vi "Labview_FFT_Linear_Tianyi.vi"(0 "Channel A":u16[](array[numeric]), 5 "Channel B":u16[](array[numeric]), 7 "Resample Array":i32[](array[numeric]), 9 "Input Parameters":T1={"Points Per A-Scan"=0, "A-Scans per B-Scan"=0, "Voltage Range"=4.0, "Card Resolution (bits)"=16}) -> (4 "Int B-Scan Channel A":sgl[][](array[numeric]), 6 "Phase B-Scan Channel A":sgl[][](array[numeric]), 10 "Int B-Scan Channel B":sgl[][](array[numeric]), 13 "Raw B":u16[][](array[numeric]), 14 "Raw A":u16[][](array[numeric]), 15 "Phase B-Scan Channel B":sgl[][](array[numeric]))   [LabVIEW 2012]
uses:
  Type Defs/OCT Imaging Parameters Cluster.ctl
  <vilib>/Analysis/4window.llb/Hanning Window (DBL).vi
  <vilib>/Analysis/2dsp.llb/Real FFT.vi
  <vilib>/Analysis/NI_AALPro.lvlib
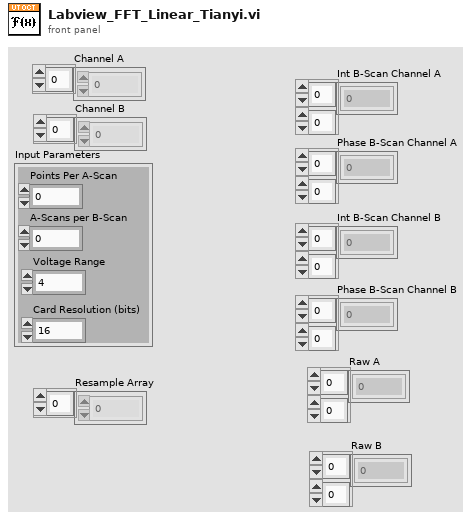
[diagram p1: front panel]
types:
  T1 = typedef "OCT Imaging Parameters Cluster.ctl" = cluster{"Points Per A-Scan":i32, "A-Scans per B-Scan":i32, "Voltage Range":sgl, "Card Resolution (bits)":u16}
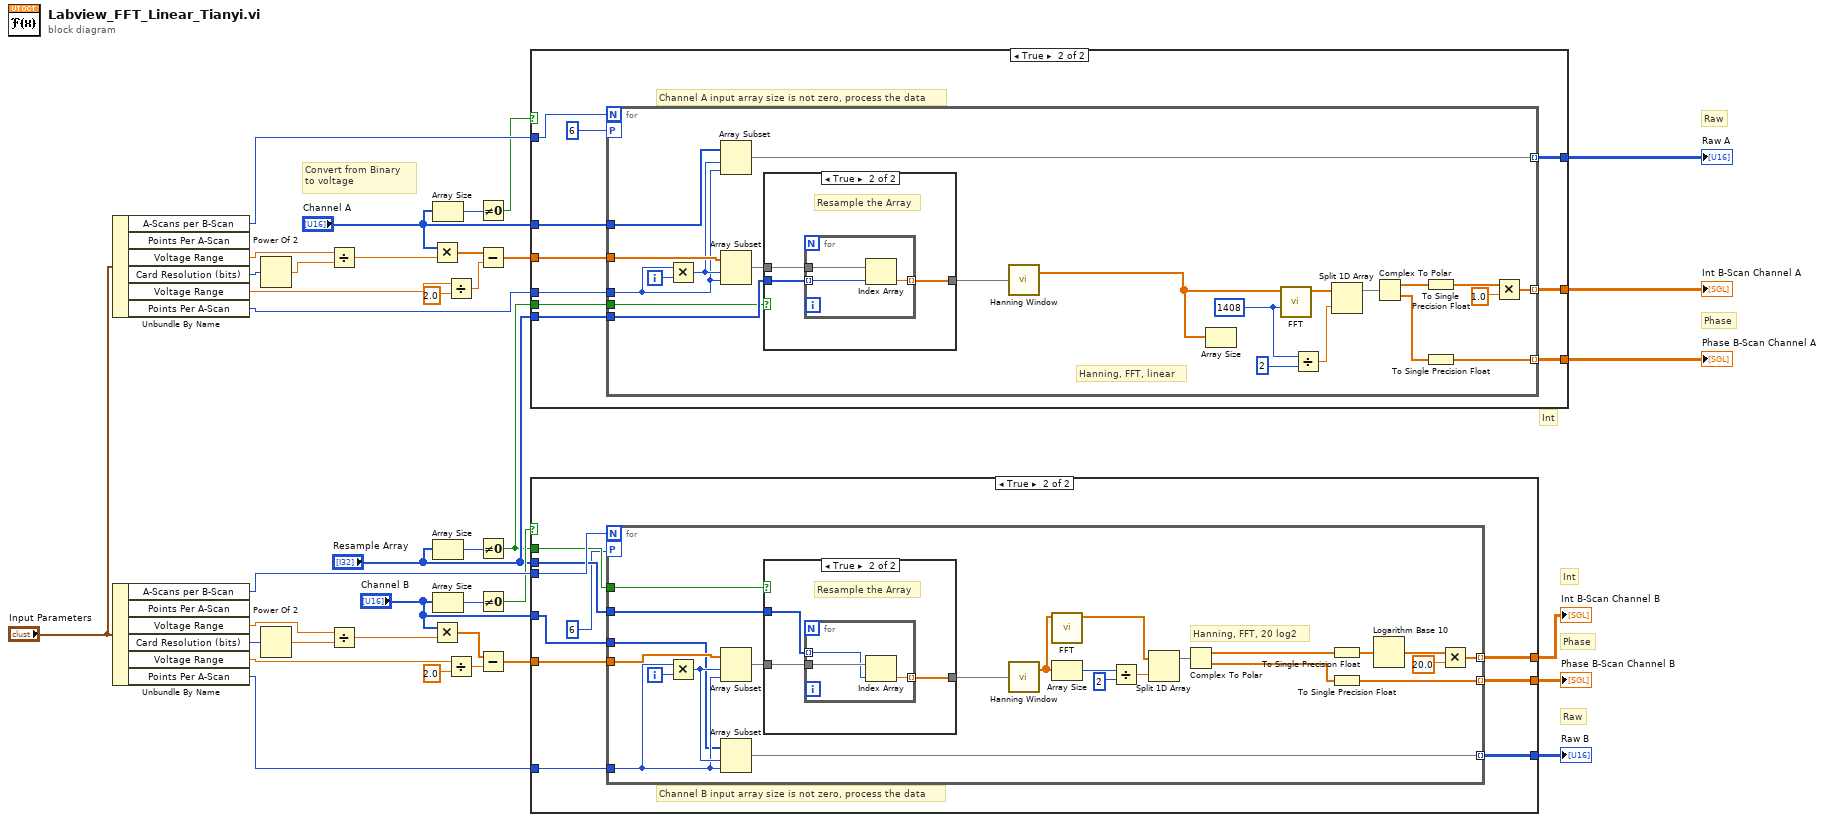
[diagram p0: block diagram]
diagram:
  # "Raw"
  # "Raw"
  # "Convert from Binary \nto voltage"
  # "Phase"
  # "Int"
  # "Phase"
  # "Int"
  n1 = Unbundle By Name("Input Parameters") -> ("A-Scans per B-Scan"=w36:i32, "Voltage Range"=w32:sgl, "Card Resolution (bits)"=w33:u16, "Voltage Range"=w30:sgl, "Points Per A-Scan"=w28:i32)  [unwired: 1 out]
  n2 = Unbundle By Name("Input Parameters") -> ("A-Scans per B-Scan"=w19:i32, "Voltage Range"=w23:sgl, "Card Resolution (bits)"=w22:u16, "Voltage Range"=w25:sgl, "Points Per A-Scan"=w27:i32)  [unwired: 1 out]
  n3 = Power Of 2(x=w33) -> (2^x=w35:dbl)
  n4 = Power Of 2(x=w22) -> (2^x=w20:dbl)
  n5 = Divide(x=w32, y=w35) -> (x/y=w34:dbl)
  n6 = Divide(x=w23, y=w20) -> (x/y=w21:dbl)
  n7 = Multiply(x="Channel A", y=w34) -> (x*y=w38:dbl[])
  n8 = Multiply(x="Channel B", y=w21) -> (x*y=w17:dbl[])
  n9 = Array Size(array="Channel A") -> (size(s)=w15:i32)
  n10 = Array Size(array="Resample Array") -> (size(s)=w3:i32)
  n11 = Array Size(array="Channel B") -> (size(s)=w13:i32)
  n12 = Divide(x=w30, y=sgl 2.0) -> (x/y=w31:sgl)
  n13 = Divide(x=w25, y=sgl 2.0) -> (x/y=w24:sgl)
  n14 = Not Equal To 0?(x=w15) -> (x != 0?=w14:bool)
  n15 = Subtract(x=w38, y=w31) -> (x-y=w37:dbl[])
  n16 = Not Equal To 0?(x=w3) -> (x != 0?=w1:bool)
  n17 = Not Equal To 0?(x=w13) -> (x != 0?=w12:bool)
  n18 = Subtract(x=w17, y=w24) -> (x-y=w18:dbl[])
  n19 = case shown="True" w14 {
    tunnel: w37 -> [_ w48]
    tunnel: [_ w47] -> w11
    tunnel: w36 -> [_ w46]
    tunnel: w28 -> [_ w45]
    tunnel: [_ w44] -> w8
    tunnel: "Channel A" -> [_ w43]
    tunnel: [_ w42] -> w6
    tunnel: "Resample Array" -> [_ w41]
    tunnel: w1 -> [_ w40]
    frame False {
      # "Channel A array size is zero, don't process data"
    }
    frame True {
      # "Channel A input array size is not zero, process the data"
      n20 = for {
        N: w46 -> [_]
        tunnel: w48 -> [w70]
        tunnel: w45 -> [w59]
        tunnel: [w66] -> w47 mode=indexing
        tunnel: [w62] -> w44 mode=indexing
        tunnel: w43 -> [w61]
        tunnel: [w58] -> w42 mode=indexing
        tunnel: w41 -> [w57]
        tunnel: w40 -> [w54]
        workers-P: 6 -> [_]
        i -> [w69]
        w49 = 1408 ("FFT size")
        # "Hanning, FFT, linear"
        n21 = Multiply(x=w59, y=w69) -> (x*y=w60:i32)
        n22 = Array Subset(array=w61, index=w60, length=w59) -> (w58:u16[])
        n23 = Array Subset(array=w70, index=w60, length=w59) -> (w56:dbl[])
        n24 = case shown="True" w54 {
          tunnel: w56 -> [w71 w74]
          tunnel: [w71 w73] -> w55
          tunnel: w57 -> [_ w72]
          frame False {
          }
          frame True {
            # "Resample the Array"
            n25 = for {
              tunnel: w72 -> [w76] mode=indexing
              tunnel: w74 -> [w77]
              tunnel: [w75] -> w73 mode=indexing
              n26 = Index Array(array=w77, index=w76) -> (element=w75:dbl)
            }
          }
        }
        n27 = call-poly <vilib>:"Hanning Window.vi"("X"=w55) -> ("Windowed X"=w50:dbl[])  [unwired: 1 out]
        n28 = Array Size(array=w50) -> ()  [unwired: 1 out]
        n29 = call-poly <vilib>:"FFT.vi"("FFT size"=w49, "X"=w50) -> ("FFT {X}"=w52:cdb[])  [unwired: 8 in, 1 out]
        n30 = Divide(x=w49, y=2) -> (x/y=w64:dbl)
        n31 = Split 1D Array(array=w52, index=w64) -> (first subarray=w51:cdb[])  [unwired: 1 out]
        n32 = Complex To Polar(r * e^(i*theta)=w51) -> (r=w68:dbl[], theta=w63:dbl[])
        n33 = To Single Precision Float(number=w68) -> (single precision float=w53:sgl[])
        n34 = To Single Precision Float(number=w63) -> (single precision float=w62:sgl[])
        n35 = Multiply(x=w53, y=sgl 1.0) -> (x*y=w66:sgl[])
      }
    }
  }
  "Int B-Scan Channel A" <- w11
  "Phase B-Scan Channel A" <- w8
  "Raw A" <- w6
  n36 = case shown="True" w12 {
    tunnel: w27 -> [_ w87]
    tunnel: w19 -> [_ w86]
    tunnel: w18 -> [_ w85]
    tunnel: [_ w84] -> w10
    tunnel: [_ w83] -> w9
    tunnel: "Channel B" -> [_ w82]
    tunnel: [_ w81] -> w4
    tunnel: "Resample Array" -> [_ w80]
    tunnel: w1 -> [_ w79]
    frame False {
      # "Channel B array size is zero, don't process data"
    }
    frame True {
      # "Channel B input array size is not zero, process the data"
      n37 = for {
        N: w86 -> [_]
        tunnel: w85 -> [w110]
        tunnel: w87 -> [w94]
        tunnel: [w103] -> w84 mode=indexing
        tunnel: [w96] -> w83 mode=indexing
        tunnel: w82 -> [w93]
        tunnel: [w92] -> w81 mode=indexing
        tunnel: w80 -> [w90]
        tunnel: w79 -> [w89]
        workers-P: 6 -> [_]
        i -> [w109]
        # "Hanning, FFT, 20 log2"
        n38 = Multiply(x=w94, y=w109) -> (x*y=w95:i32)
        n39 = Array Subset(array=w110, index=w95, length=w94) -> (w91:dbl[])
        n40 = Array Subset(array=w93, index=w95, length=w94) -> (w92:u16[])
        n41 = case shown="True" w89 {
          tunnel: w91 -> [w111 w114]
          tunnel: [w111 w113] -> w88
          tunnel: w90 -> [_ w112]
          frame False {
          }
          frame True {
            # "Resample the Array"
            n42 = for {
              tunnel: w112 -> [w116] mode=indexing
              tunnel: w114 -> [w117]
              tunnel: [w115] -> w113 mode=indexing
              n43 = Index Array(array=w117, index=w116) -> (element=w115:dbl)
            }
          }
        }
        n44 = call-poly <vilib>:"Hanning Window.vi"("X"=w88) -> ("Windowed X"=w101:dbl[])  [unwired: 1 out]
        n45 = call-poly <vilib>:"FFT.vi"("X"=w101) -> ("FFT {X}"=w102:cdb[])  [unwired: 9 in, 1 out]
        n46 = Array Size(array=w101) -> (size(s)=w100:i32)
        n47 = Divide(x=w100, y=2) -> (x/y=w98:dbl)
        n48 = Split 1D Array(array=w102, index=w98) -> (first subarray=w108:cdb[])  [unwired: 1 out]
        n49 = Complex To Polar(r * e^(i*theta)=w108) -> (r=w107:dbl[], theta=w97:dbl[])
        n50 = To Single Precision Float(number=w107) -> (single precision float=w106:sgl[])
        n51 = To Single Precision Float(number=w97) -> (single precision float=w96:sgl[])
        n52 = Logarithm Base 10(1:w106) -> (0:w105:sgl[])
        n53 = Multiply(x=w105, y=sgl 20.0) -> (x*y=w103:sgl[])
      }
    }
  }
  "Int B-Scan Channel B" <- w10
  "Phase B-Scan Channel B" <- w9
  "Raw B" <- w4
